vi "CPLX_DBL.vi"(4 "Value":cdb) -> (1 "Constant":refnum<class "Abs_Complex Double Float.lvclass">)   [LabVIEW 2021, in "Const_CPLX_DBL.lvclass"]
uses:
  Const_CPLX_DBL.lvclass
  Abs_Types/Complex Double Float/Abs_Complex Double Float.lvclass
  C:/Program Files (x86)/National Instruments/LabVIEW 2021/vi.lib/TSA/Abstract Data Classes/Abs_Types/Complex Double Float/Abs_Complex Double Float.lvclass
  Const_CPLX_DBL.lvclass/Const_CPLX_DBL.ctl
  Properties/Write Value.vi
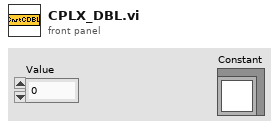
[diagram p1: front panel]
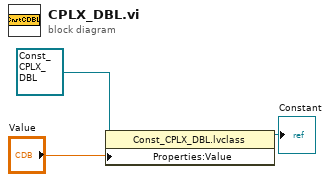
[diagram p0: block diagram]
diagram:
  n1 = property class="Const_CPLX_DBL.lvclass"(reference=refnum<class "Const_CPLX_DBL.lvclass"> refnum ("Constants.lvlib:Numeric.lvclass"), "Properties:Value"="Value") -> (reference out=→"Constant":refnum<class "Const_CPLX_DBL.lvclass">)  [unwired: 1 in, 1 out]
